vi "QuickDrop Toggle probe.vi"(6 "Variant in":variant, 7 "Shift Pressed?":bool, 8 "error in (no error)":errorcluster, 10 "QD Combo Box Ref":refnum<vi>, 11 "QD Launch VI Ref":refnum<vi>) -> (0 "error out":errorcluster, 4 "Variant out":variant)   [LabVIEW 2022 SP3]
doc: "<b>Quick drop box tool:</b> toggles probes on the selected wires. If this function is called with the shift selected then it also toggles breakpoints.\n\nDefault Shortcut - [V]"
uses:
  <vilib>/Utility/miscctls.llb/LVBreakpointStatusEnum.ctl
panel:
  in  "Undo Name":string="Create Inputs and/or Outputs"
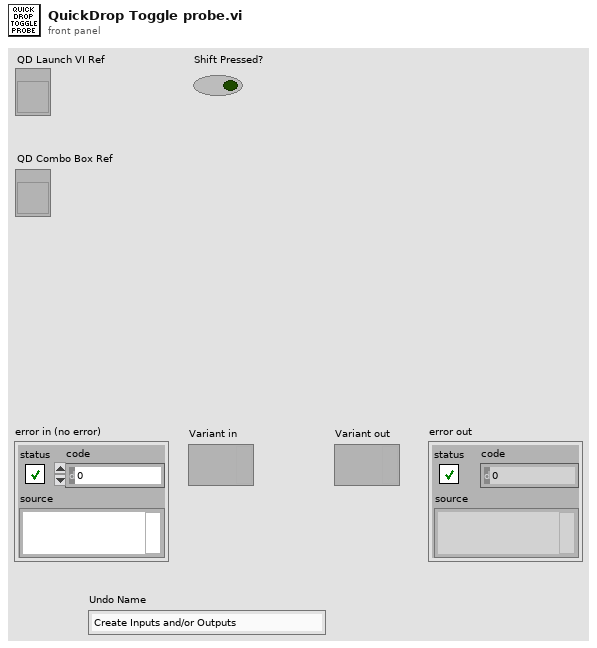
[diagram p1: front panel]
types:
  T1 = typedef "LVBreakpointStatusEnum.ctl" = enum8{"Cleared Break", "Enabled Break", "Disabled Break"}
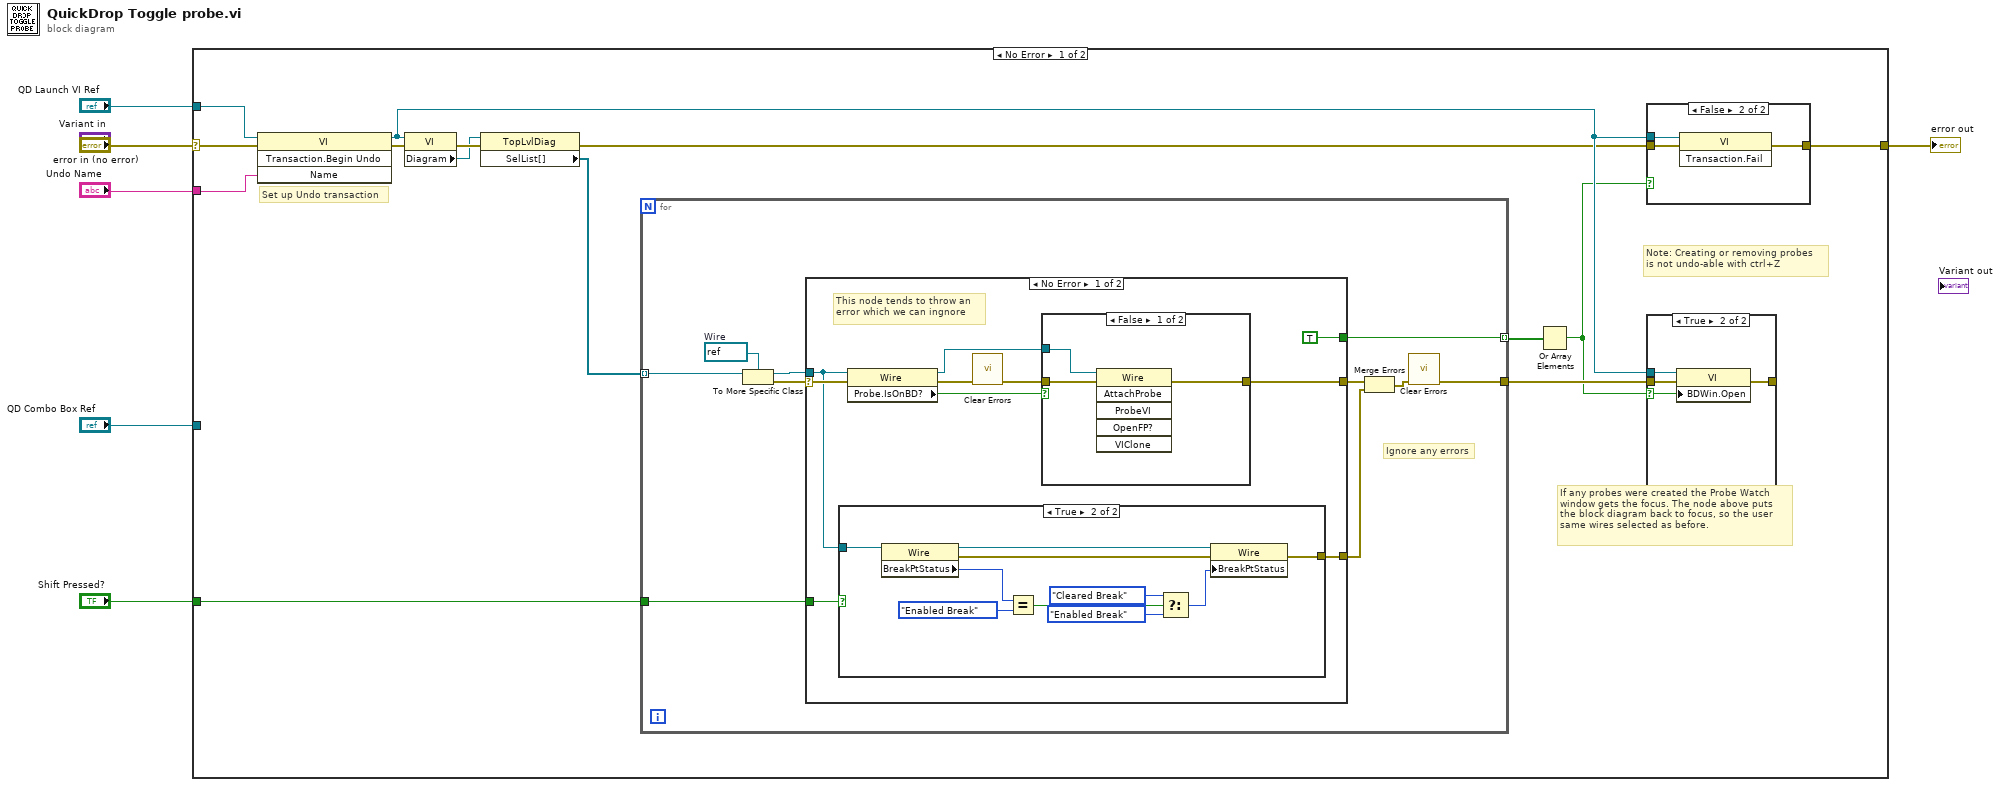
[diagram p0: block diagram]
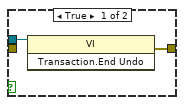
[diagram p2: hidden frame]
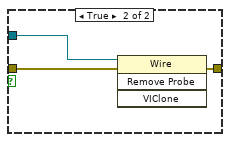
[diagram p3: hidden frame]
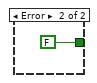
[diagram p5: hidden frame]
diagram:
  n1 = case shown="No Error" "error in (no error)" {
    selector: "error in (no error)" -> [w20 w67]
    tunnel: [w8 w67] -> w5
    tunnel: "Shift Pressed?" -> [w11 _]
    tunnel: "QD Combo Box Ref" -> [_ _]
    tunnel: "QD Launch VI Ref" -> [w15 _]
    tunnel: "Undo Name" -> [w17 _]
    frame No Error {
      # "Note: Creating or removing probes\nis not undo-able with ctrl+Z"
      # "If any probes were created the Probe Watch\nwindow gets the focus. The node above puts\nthe block diagram back to focus, so the user\nsame wires selected as before."
      # "Set up Undo transaction"
      n2 = invoke class="VI" method="Transaction.Begin Undo"(reference=w15, error in=w20, "Name"=w17) -> (reference out=w10:refnum<vi>, error out=w18:errorcluster)  [unwired: 1 in, 2 out]
      n3 = property class="VI"(reference=w10, error in=w18) -> (error out=w19:errorcluster, "Diagram"=w14:refnum<vi>)  [unwired: 1 out]
      n4 = property class="TopLvlDiag"(reference=w14, error in=w19) -> (error out=w7:errorcluster, "SelList[]"=w16:refnum<vi>[])  [unwired: 1 out]
      n5 = for {
        tunnel: w16 -> [w31] mode=indexing
        tunnel: [w30] -> w13
        tunnel: [w29] -> w12 mode=indexing
        tunnel: w11 -> [w28]
        w35 = refnum<vi> refnum  # Wire
        # "Ignore any errors"
        n6 = To More Specific Class(target class=w35, reference=w31) -> (specific class reference=w33:refnum<vi>, error out=w34:errorcluster)  [unwired: 1 in]
        n7 = case shown="No Error" w34 {
          selector: w34 -> [w44 _]
          tunnel: w33 -> [w37 _]
          tunnel: [w45 _] -> w32
          tunnel: [TRUE FALSE] -> w29
          tunnel: w28 -> [w38 _]
          tunnel: [w36 _] -> w26
          frame No Error {
            # "This node tends to throw an \nerror which we can ingnore"
            n8 = case shown="True" w38 {
              tunnel: w37 -> [_ w53]
              tunnel: [_ w52] -> w36
              frame False {
              }
              frame True {
                n9 = property class="Wire"(reference=w53) -> (reference out=w61:refnum<vi>, error out=w58:errorcluster, "BreakPtStatus"=w57:T1)  [unwired: 1 in]
                n10 = Equal?(x=w57, y=LVBreakpointStatusEnum."Enabled Break") -> (x = y?=w59:bool)
                n11 = Select(t=LVBreakpointStatusEnum."Cleared Break", s=w59, f=LVBreakpointStatusEnum."Enabled Break") -> (s? t:f=w60:T1)
                n12 = property class="Wire"(reference=w61, error in=w58, "BreakPtStatus"=w60) -> (error out=w52:errorcluster)  [unwired: 1 out]
              }
            }
            n13 = property class="Wire"(reference=w37, error in=w44) -> (reference out=w40:refnum<vi>, error out=w41:errorcluster, "Probe.IsOnBD?"=w43:bool)
            n14 = call <vilib>:"Clear Errors.vi"("error in (no error)"=w41) -> ("error out"=w42:errorcluster)  [unwired: 5 in, 1 out]
            n15 = case shown="False" w43 {
              tunnel: [w46 w49] -> w45
              tunnel: w40 -> [w48 w50]
              tunnel: w42 -> [w47 w51]
              frame False {
                n16 = invoke class="Wire" method="AttachProbe"(reference=w48, error in=w47) -> (error out=w46:errorcluster)  [unwired: 4 in, 5 out]
              }
              frame True {
                n17 = invoke class="Wire" method="Remove Probe"(reference=w50, error in=w51) -> (error out=w49:errorcluster)  [unwired: 2 in, 3 out]
              }
            }
          }
          frame Error {
          }
        }
        n18 = Merge Errors(w32, w26) -> (w27:errorcluster)
        n19 = call <vilib>:"Clear Errors.vi"("error in (no error)"=w27) -> ("error out"=w30:errorcluster)  [unwired: 5 in, 1 out]
      }
      n20 = Or Array Elements(Boolean array=w12) -> (logical OR=w9:bool)
      n21 = case shown="False" w9 {
        tunnel: w10 -> [w21 w24]
        tunnel: [w22 w25] -> w8
        tunnel: w7 -> [_ w23]
        frame True {
          n22 = invoke class="VI" method="Transaction.End Undo"(reference=w21) -> (error out=w22:errorcluster)  [unwired: 2 in, 2 out]
        }
        frame False {
          n23 = invoke class="VI" method="Transaction.Fail"(reference=w24, error in=w23) -> (error out=w25:errorcluster)  [unwired: 1 in, 2 out]
        }
      }
      n24 = case shown="True" w9 {
        selector: w9 -> [_ w64]
        tunnel: w13 -> [_ w66]
        tunnel: w10 -> [_ w65]
        tunnel: [_ w63] -> _
        frame False {
        }
        frame True {
          n25 = property class="VI"(reference=w65, error in=w66, "BDWin.Open"=w64) -> (error out=w63:errorcluster)  [unwired: 1 out]
        }
      }
    }
    frame Error {
    }
  }
  "error out" <- w5
